vi "Test v2 Client.vi"() -> ()   [LabVIEW 2020, in "InfluxDB v2 Client.lvlib"]
uses:
  InfluxDB v2 Client.lvlib
  Client/Header-Body Data.ctl
  Client/Error Handler/HTTP Status.ctl
  Client/DataBase Data.ctl
  Data Point/Tag.ctl
  Field Values.ctl
  Client/Write Data.ctl
  Client/Write Precision.ctl
  Client/Influx Command.ctl
  Setup/Setup Data.ctl
  Data Point/Data Point - Cmd.ctl
  <vilib>/Utility/xml.llb/Read From XML File(string).vi
  <vilib>/Utility/xml.llb/Write to XML File(string).vi
panel:
  out "Response":T1
  in  "Tab Control":enum32{"Setup", "Init", "Write", "Query"}(tab)
  in  "Write Setup":bool
  in  "Read Setup":bool
  in  "File Path Setup":path
  in  "Init":bool
  in  "Check Auth":bool
  in  "DataBase Data":T2
  in  "Init Write Data":bool
  in  "Write Data":bool
  in  "Field Names":string[](array[string])=["cpu_temp", "error_code", "cpu_load", "cpu_type", "cpu_busy"]
  in  "Tags":T3[](array[typedef])=[{"Key"="host1", "Value"="myPC"}, {"Key"="host2", "Value"="X-Server"}]
  in  "Field Values":T4={"cpu_temp"=48.25, "error_code"=-9003, "cpu_load"=8, "cpu_type"="Ryzen 5 2600", "cpu_busy?"=FALSE}
  in  "Write Data":T5={"Bucket"="", "Timestamp precision"=enum."Seconds", "Line protocol"="", "Measurement"=""}
  in  "Write Query":bool
  in  "Read Query":bool
  in  "with compression?":bool
  in  "Write csv - file":bool
  in  "Query":string="from(bucket: \"Test\")\n  |> range(start: -30m)\n  |> filter(fn: (r) => r[\"_measurement\"] == \"mem3\")\n  |> filter(fn: (r) => r[\"_field\"] == \"cpu_temp\")\n  |> aggregateWindow(every: 1s, fn: last, createEmpty: false)\n  |> yield(name: \"last\")"
  in  "Query Data":bool
  in  "File Path Queries":path
  out "HTTP Status":T7
  in  "Stop":bool
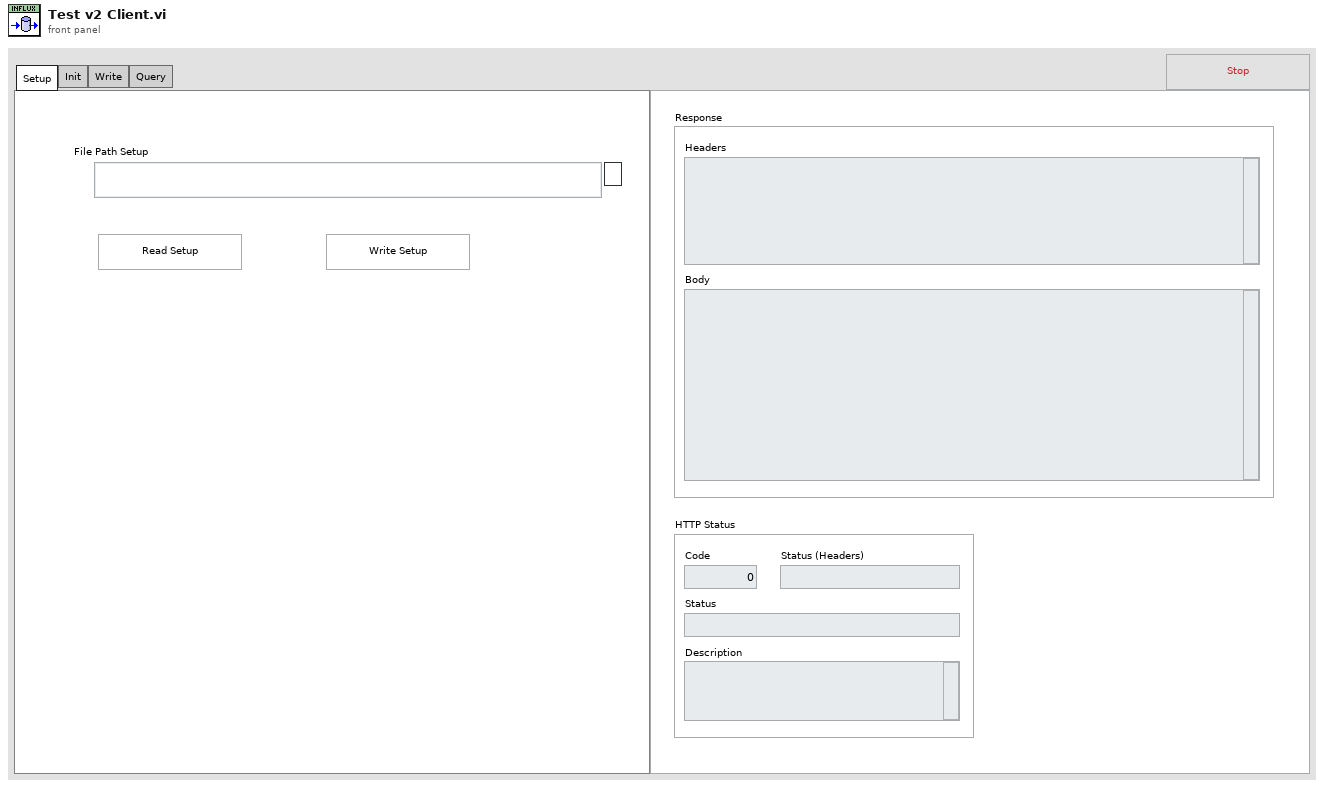
[diagram p1: front panel]
types:
  T1 = typedef "InfluxDB v2 Client.lvlib/Header-Body Data.ctl" = cluster{"Headers":string, "Body":string}
  T2 = typedef "InfluxDB v2 Client.lvlib/DataBase Data.ctl" = cluster{"Api Token":string, "Organization":string, "url":string, "Organization ID":string}
  T3 = typedef "InfluxDB v2 Client.lvlib/Tag.ctl" = cluster{"Key":string, "Value":string}
  T4 = typedef "InfluxDB v2 Client.lvlib/Field Values.ctl" = cluster{"cpu_temp":dbl, "error_code":i64, "cpu_load":u64, "cpu_type":string, "cpu_busy?":bool}
  T5 = typedef "InfluxDB v2 Client.lvlib/Write Data.ctl" = cluster{"Bucket":string, "Timestamp precision":T6, "Line protocol":string, "Measurement":string}
  T6 = typedef "InfluxDB v2 Client.lvlib/Write Precision.ctl" = enum16{"Nanoseconds", "Microseconds", "Milliseconds", "Seconds"}
  T7 = typedef "InfluxDB v2 Client.lvlib/HTTP Status.ctl" = cluster{"Code":i32, "Status":string, "Description":string, "Status (Headers)":string}
  T8 = typedef "InfluxDB v2 Client.lvlib/Influx Command.ctl" = enum16{"Init", "Check Auth", "Query Data", "Query ZIP Data", "Write Data", "Close"}
  T9 = enum16{"open", "replace", "create", "open or create", "replace or create", "replace or create with confirmation"}
  T10 = typedef "InfluxDB v2 Client.lvlib/Data Point - Cmd.ctl" = enum16{"Init", "Add Tags", "Add Fields", "Add Field Names", "Add Field Values", "Add Measurement", "Add Time Stamp", "Add Precision", "Get Line Protocol"}
  T11 = typedef "InfluxDB v2 Client.lvlib/Setup Data.ctl" = cluster{"DataBase Data":T2, "Write Data":T5, "Query - csv":string}
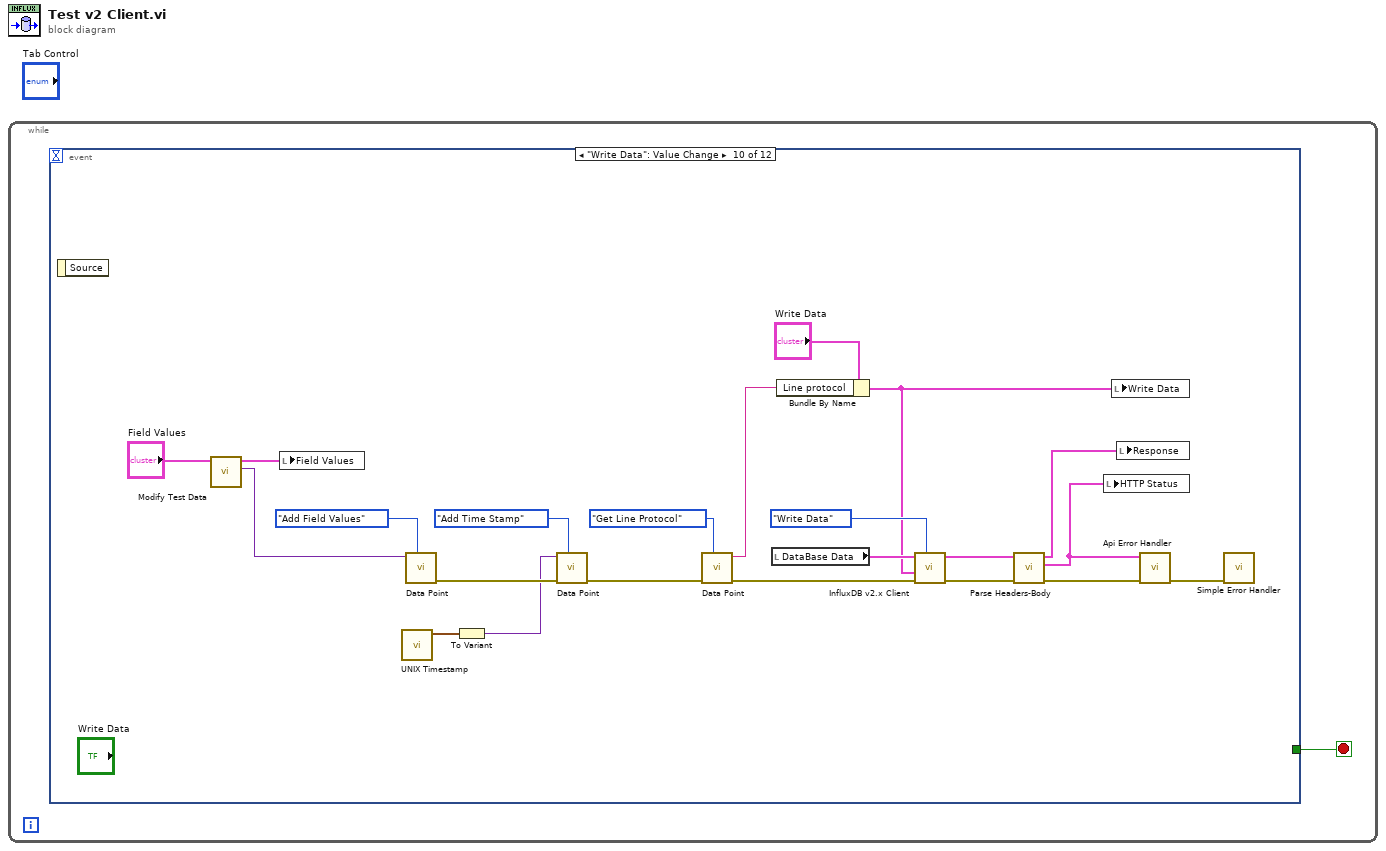
[diagram p0: block diagram]
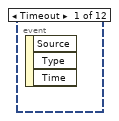
[diagram p2: hidden frame]
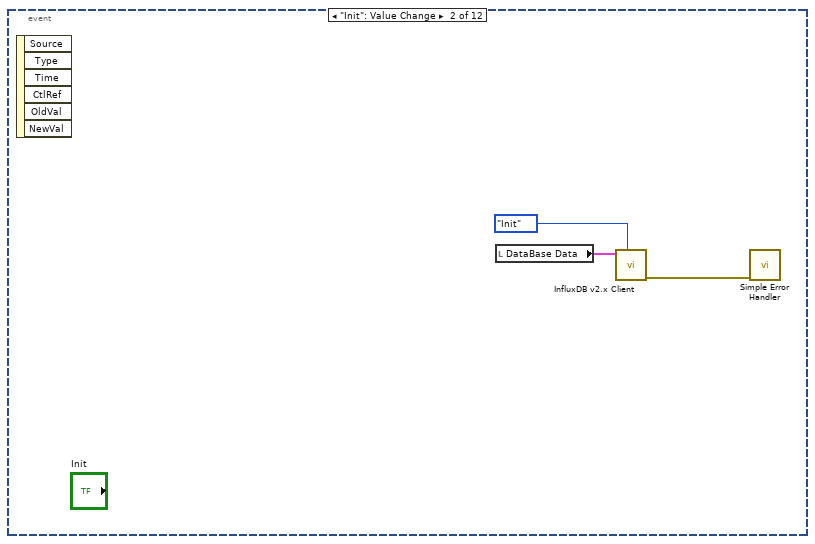
[diagram p3: hidden frame]
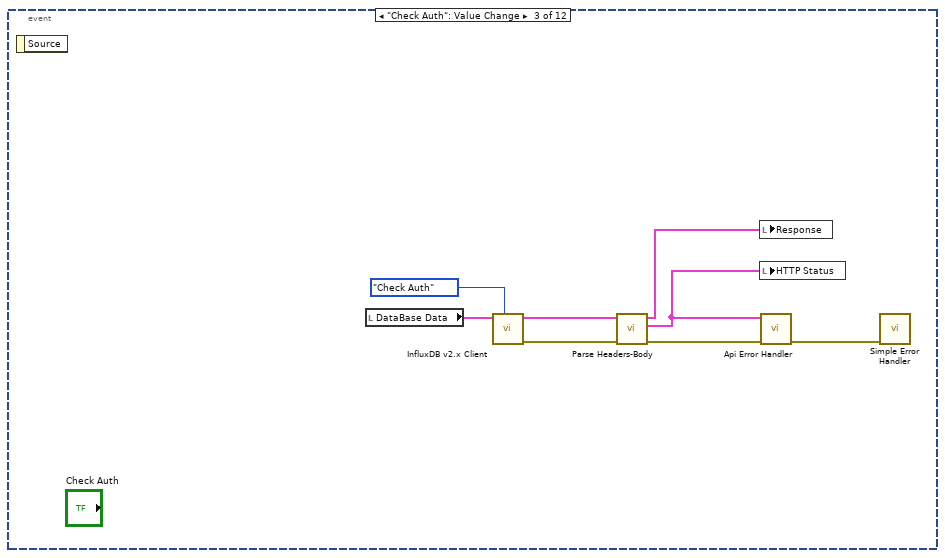
[diagram p4: hidden frame]
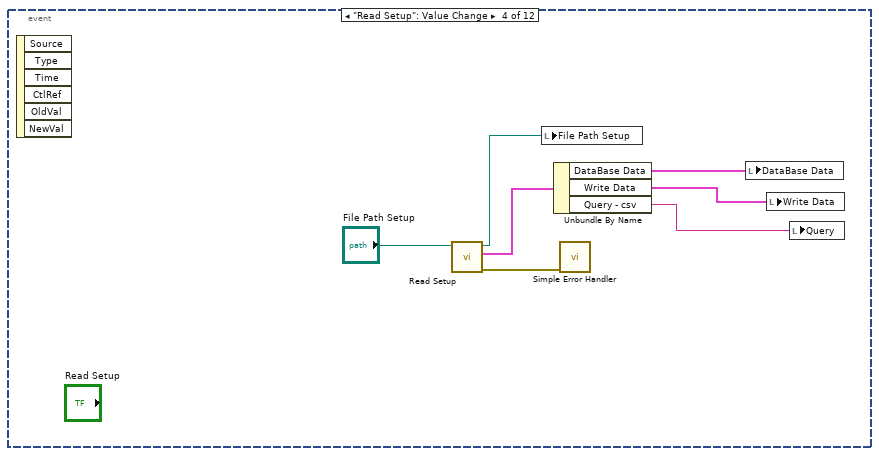
[diagram p5: hidden frame]
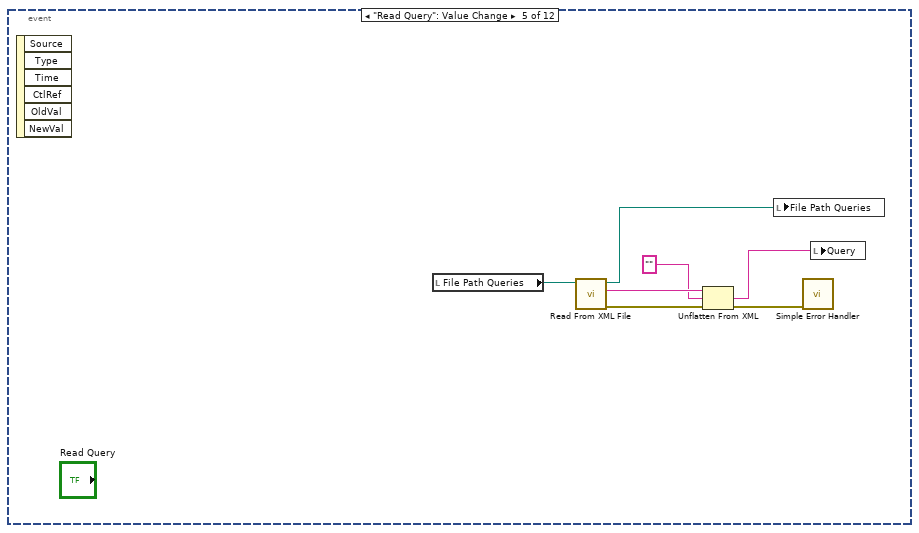
[diagram p6: hidden frame]
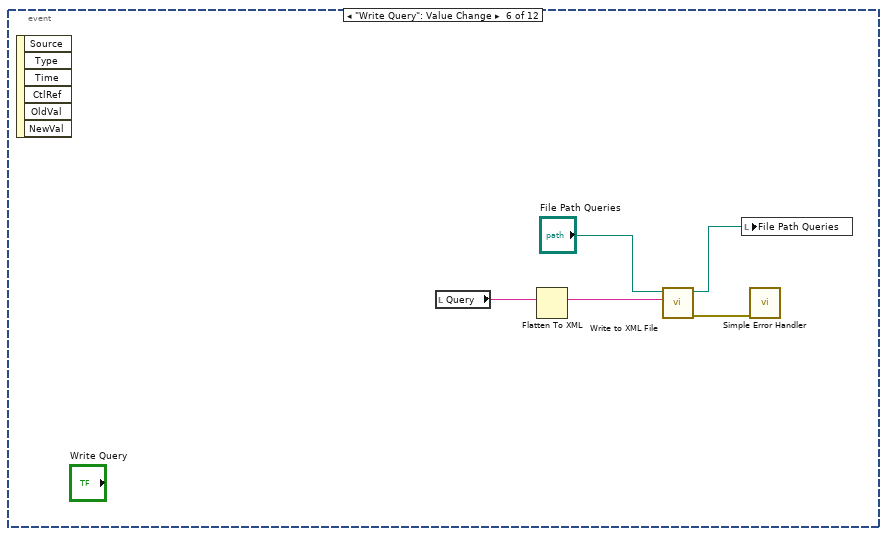
[diagram p7: hidden frame]
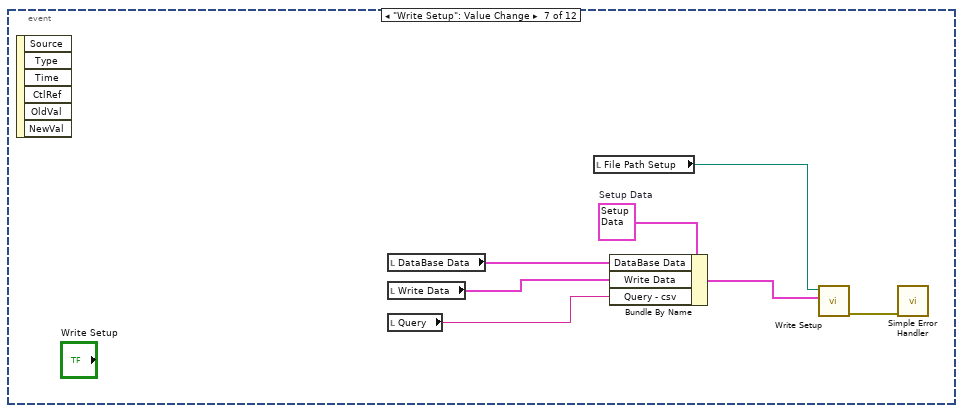
[diagram p8: hidden frame]
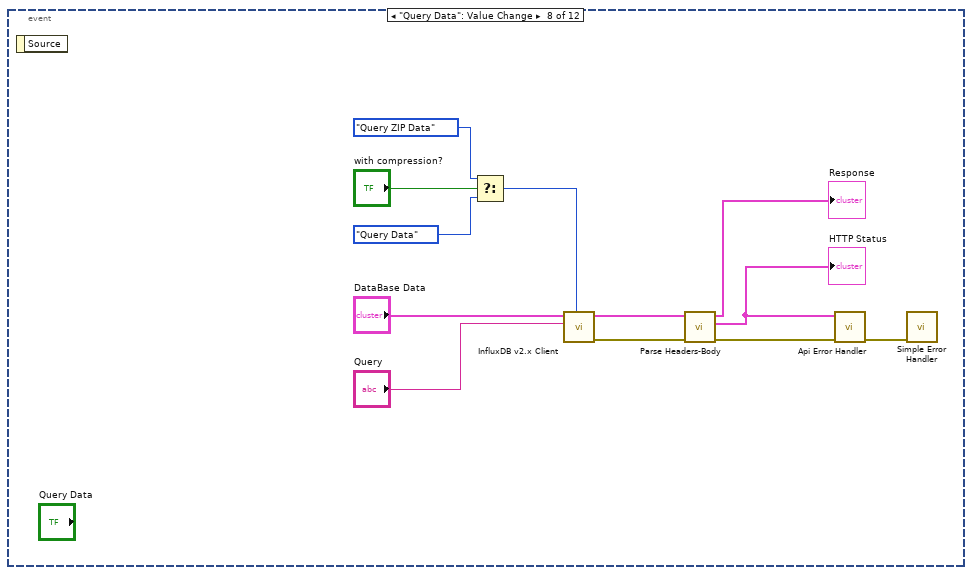
[diagram p9: hidden frame]
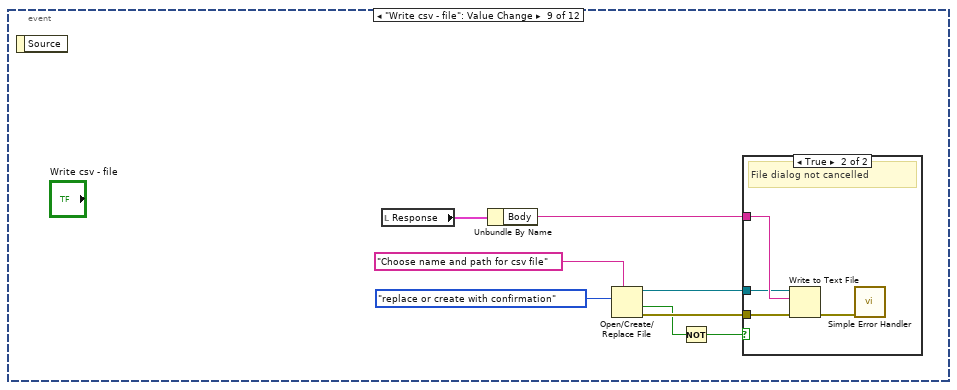
[diagram p10: hidden frame]
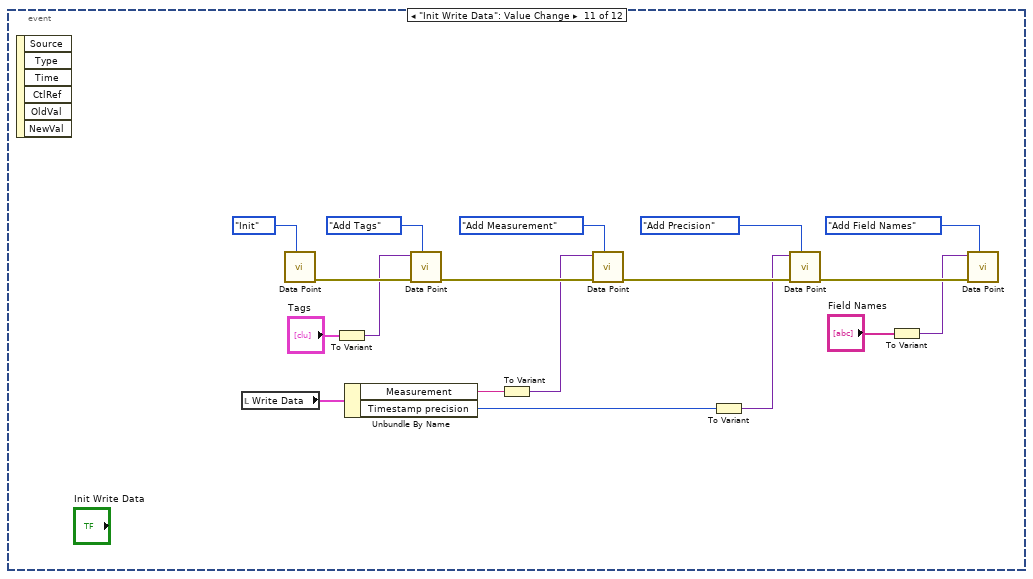
[diagram p12: hidden frame]
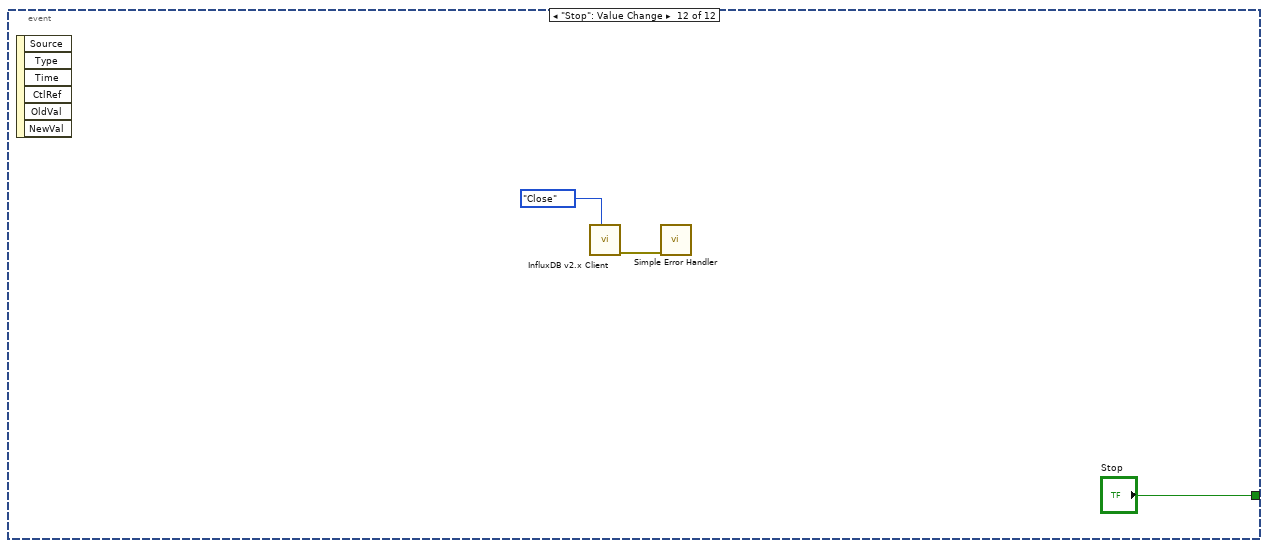
[diagram p13: hidden frame]
diagram:
  n1 = while {
    stop <- w1 stop-if-true
    n2 = event shown="[9] \"Write Data\": Value Change" {
      selector: _ -> [_ _ _ _ _ _ _ _ _ _ _ _]
      dyn-events: _ -> [_ _ _ _ _ _ _ _ _ _ _ _]
      timeout: _ -> [_ _ _ _ _ _ _ _ _ _ _ _]
      tunnel: [_ _ _ _ _ _ _ _ _ _ _ "Stop"] -> w1
      event Timeout {
        n3 = event-data() -> ()  [unwired: 1 in, 3 out]
      }
      event "Init": Value Change {
        n4 = event-data() -> ()  [unwired: 1 in, 6 out]
        n5 = local read "DataBase Data"() -> (w2:T2)
        n6 = call "InfluxDB v2.x Client.vi"("Influx Command"=Influx_Command."Init", "DataBase Data"=w2) -> ("error out"=w3:errorcluster)  [unwired: 8 in, 1 out]
        n7 = call <vilib>:"Simple Error Handler.vi"("error in (no error)"=w3) -> ()  [unwired: 4 in, 5 out]
      }
      event "Check Auth": Value Change {
        n8 = event-data() -> ()  [unwired: 1 in, 1 out]
        n9 = local read "DataBase Data"() -> (w10:T2)
        n10 = call "InfluxDB v2.x Client.vi"("Influx Command"=Influx_Command."Check Auth", "DataBase Data"=w10) -> ("error out"=w9:errorcluster, "Header-Body Data"=w7:T1)  [unwired: 8 in]
        n11 = call "Parse Headers-Body.vi"("error in"=w9, "Header-Body Data in"=w7) -> ("error out"=w8:errorcluster, "HTTP Status"=w5:T7, "Header-Body Data out"=w6:T1)  [unwired: 7 in]
        n12 = local write "Response"(w6) -> ()
        n13 = local write "HTTP Status"(w5) -> ()
        n14 = call "Api Error Handler.vi"("error in"=w8, "HTTP Status"=w5) -> ("error out"=w11:errorcluster)  [unwired: 9 in]
        n15 = call <vilib>:"Simple Error Handler.vi"("error in (no error)"=w11) -> ()  [unwired: 4 in, 5 out]
      }
      event "Read Setup": Value Change {
        n16 = event-data() -> ()  [unwired: 1 in, 6 out]
        n17 = call "Read Setup.vi"("File Path in"="File Path Setup") -> ("error out"=w16:errorcluster, "Setup Data"=w15:T11, "File Path out"=w14:path)  [unwired: 8 in]
        n18 = local write "File Path Setup"(w14) -> ()
        n19 = Unbundle By Name(w15) -> ("DataBase Data"=w18:T2, "Write Data"=w13:T5, "Query - csv"=w17:string)
        n20 = call <vilib>:"Simple Error Handler.vi"("error in (no error)"=w16) -> ()  [unwired: 4 in, 5 out]
        n21 = local write "DataBase Data"(w18) -> ()
        n22 = local write "Write Data"(w13) -> ()
        n23 = local write "Query"(w17) -> ()
      }
      event "Read Query": Value Change {
        n24 = event-data() -> ()  [unwired: 1 in, 6 out]
        n25 = local read "File Path Queries"() -> (w26:path)
        n26 = call-poly <vilib>:"Read From XML File.vi"("XML File Path"=w26) -> ("error out"=w24:errorcluster, "XML Elements"=w23:string, "XML File Path(duplicate)"=w25:path)  [unwired: 8 in]
        n27 = Unflatten From XML(xml string=w23, type="", error in (no error)=w24) -> (value=w21:string, error out=w20:errorcluster)
        n28 = local write "File Path Queries"(w25) -> ()
        n29 = call <vilib>:"Simple Error Handler.vi"("error in (no error)"=w20) -> ()  [unwired: 4 in, 5 out]
        n30 = local write "Query"(w21) -> ()
      }
      event "Write Query": Value Change {
        n31 = event-data() -> ()  [unwired: 1 in, 6 out]
        n32 = local read "Query"() -> (w31:string)
        n33 = Flatten To XML(6:w31) -> (2:w30:string)
        n34 = call-poly <vilib>:"Write to XML File.vi"("XML Input"=w30, "XML File Path"="File Path Queries") -> ("error out"=w27:errorcluster, "XML File Path(duplicate)"=w28:path)  [unwired: 7 in, 1 out]
        n35 = local write "File Path Queries"(w28) -> ()
        n36 = call <vilib>:"Simple Error Handler.vi"("error in (no error)"=w27) -> ()  [unwired: 4 in, 5 out]
      }
      event "Write Setup": Value Change {
        w38 = T11 {"DataBase Data"={"Api Token"="", "Organization"="", "url"="", "Organization ID"=""}, "Write Data"={"Bucket"="", "Timestamp precision"=enum."Seconds", "Line protocol"="", "Measurement"=""}, "Query - csv"=""}  # Setup Data
        n37 = event-data() -> ()  [unwired: 1 in, 6 out]
        n38 = local read "DataBase Data"() -> (w37:T2)
        n39 = local read "Write Data"() -> (w32:T5)
        n40 = local read "Query"() -> (w36:string)
        n41 = local read "File Path Setup"() -> (w35:path)
        n42 = Bundle By Name(cluster=w38, "DataBase Data"=w37, "Write Data"=w32, "Query - csv"=w36) -> (w34:T11)
        n43 = call "Write Setup.vi"("Setup Data"=w34, "File Path"=w35) -> ("error out"=w33:errorcluster)  [unwired: 9 in]
        n44 = call <vilib>:"Simple Error Handler.vi"("error in (no error)"=w33) -> ()  [unwired: 4 in, 5 out]
      }
      event "Query Data": Value Change {
        n45 = event-data() -> ()  [unwired: 1 in, 1 out]
        n46 = Select(t=Influx_Command."Query ZIP Data" ("Influx Command"), s="with compression?", f=Influx_Command."Query Data" ("Influx Command")) -> (s? t:f=w44:T8)
        n47 = call "InfluxDB v2.x Client.vi"("Influx Command"=w44, "Query Data"="Query", "DataBase Data"="DataBase Data") -> ("error out"=w43:errorcluster, "Header-Body Data"=w42:T1)  [unwired: 7 in]
        n48 = call "Parse Headers-Body.vi"("error in"=w43, "Header-Body Data in"=w42) -> ("error out"=w41:errorcluster, "HTTP Status"=w39:T7, "Header-Body Data out"=→"Response":T1)  [unwired: 7 in]
        "HTTP Status" <- w39
        n49 = call "Api Error Handler.vi"("error in"=w41, "HTTP Status"=w39) -> ("error out"=w50:errorcluster)  [unwired: 9 in]
        n50 = call <vilib>:"Simple Error Handler.vi"("error in (no error)"=w50) -> ()  [unwired: 4 in, 5 out]
      }
      event "Write csv - file": Value Change {
        n51 = event-data() -> ()  [unwired: 1 in, 1 out]
        n52 = local read "Response"() -> (w58:T1)
        n53 = Unbundle By Name(w58) -> ("Body"=w57:string)
        n54 = Open/Create/Replace File(prompt="Choose name and path for csv file" ("prompt (Choose or enter file path)"), operation (0:open)=T9."replace or create with confirmation") -> (refnum out=w53:refnum<file>, cancelled=w52:bool, error out=w54:errorcluster)  [unwired: 4 in]
        n55 = Not(x=w52) -> (.not. x?=w51:bool)
        n56 = case shown="True" w51 {
          tunnel: w57 -> [_ w62]
          tunnel: w54 -> [_ w61]
          tunnel: w53 -> [_ w60]
          frame False {
          }
          frame True {
            # "File dialog not cancelled"
            n57 = Write to Text File(file (use dialog)=w60, text=w62, error in=w61) -> (error out=w59:errorcluster)  [unwired: 1 in, 2 out]
            n58 = call <vilib>:"Simple Error Handler.vi"("error in (no error)"=w59) -> ()  [unwired: 4 in, 5 out]
          }
        }
      }
      event "Write Data": Value Change {
        n59 = event-data() -> ()  [unwired: 1 in, 1 out]
        n60 = call "Modify Test Data.vi"("Field Values in"="Field Values") -> ("Variant"=w70:variant, "Field Values out"=w71:T4)  [unwired: 9 in]
        n61 = local write "Field Values"(w71) -> ()
        n62 = call "UNIX Timestamp.vi"() -> ("UNIX Time Stamp"=w74:timestamp)  [unwired: 11 in]
        n63 = call "Data Point.vi"("Data Point - Cmd"=Data_Point_-_Cmd."Add Field Values", "Data"=w70) -> ("error out"=w78:errorcluster)  [unwired: 8 in, 1 out]
        n64 = To Variant(anything=w74) -> (Variant=w75:variant)
        n65 = call "Data Point.vi"("Data Point - Cmd"=Data_Point_-_Cmd."Add Time Stamp", "error in"=w78, "Data"=w75) -> ("error out"=w76:errorcluster)  [unwired: 7 in, 1 out]
        n66 = call "Data Point.vi"("Data Point - Cmd"=Data_Point_-_Cmd."Get Line Protocol", "error in"=w76) -> ("error out"=w73:errorcluster, "Line protocol"=w80:string)  [unwired: 8 in]
        n67 = local read "DataBase Data"() -> (w82:T2)
        n68 = Bundle By Name(cluster="Write Data", "Line protocol"=w80) -> (w63:T5)
        n69 = call "InfluxDB v2.x Client.vi"("Influx Command"=Influx_Command."Write Data", "error in"=w73, "Write Data"=w63, "DataBase Data"=w82) -> ("error out"=w69:errorcluster, "Header-Body Data"=w67:T1)  [unwired: 6 in]
        n70 = call "Parse Headers-Body.vi"("error in"=w69, "Header-Body Data in"=w67) -> ("error out"=w68:errorcluster, "HTTP Status"=w65:T7, "Header-Body Data out"=w66:T1)  [unwired: 7 in]
        n71 = local write "HTTP Status"(w65) -> ()
        n72 = local write "Write Data"(w63) -> ()
        n73 = local write "Response"(w66) -> ()
        n74 = call "Api Error Handler.vi"("error in"=w68, "HTTP Status"=w65) -> ("error out"=w83:errorcluster)  [unwired: 9 in]
        n75 = call <vilib>:"Simple Error Handler.vi"("error in (no error)"=w83) -> ()  [unwired: 4 in, 5 out]
      }
      event "Init Write Data": Value Change {
        n76 = event-data() -> ()  [unwired: 1 in, 6 out]
        n77 = local read "Write Data"() -> (w87:T5)
        n78 = call "Data Point.vi"("Data Point - Cmd"=Data_Point_-_Cmd."Init") -> ("error out"=w101:errorcluster)  [unwired: 9 in, 1 out]
        n79 = To Variant(anything="Tags") -> (Variant=w98:variant)
        n80 = Unbundle By Name(w87) -> ("Measurement"=w86:string, "Timestamp precision"=w85:T6)
        n81 = call "Data Point.vi"("Data Point - Cmd"=Data_Point_-_Cmd."Add Tags", "error in"=w101, "Data"=w98) -> ("error out"=w97:errorcluster)  [unwired: 7 in, 1 out]
        n82 = To Variant(anything=w86) -> (Variant=w95:variant)
        n83 = call "Data Point.vi"("Data Point - Cmd"=Data_Point_-_Cmd."Add Measurement", "error in"=w97, "Data"=w95) -> ("error out"=w94:errorcluster)  [unwired: 7 in, 1 out]
        n84 = To Variant(anything=w85) -> (Variant=w92:variant)
        n85 = call "Data Point.vi"("Data Point - Cmd"=Data_Point_-_Cmd."Add Precision", "error in"=w94, "Data"=w92) -> ("error out"=w91:errorcluster)  [unwired: 7 in, 1 out]
        n86 = To Variant(anything="Field Names") -> (Variant=w88:variant)
        n87 = call "Data Point.vi"("Data Point - Cmd"=Data_Point_-_Cmd."Add Field Names", "error in"=w91, "Data"=w88) -> ()  [unwired: 7 in, 2 out]
      }
      event "Stop": Value Change {
        n88 = event-data() -> ()  [unwired: 1 in, 6 out]
        n89 = call "InfluxDB v2.x Client.vi"("Influx Command"=Influx_Command."Close") -> ("error out"=w103:errorcluster)  [unwired: 9 in, 1 out]
        n90 = call <vilib>:"Simple Error Handler.vi"("error in (no error)"=w103) -> ()  [unwired: 4 in, 5 out]
      }
    }
  }
